vi "run.description.vi"(8 "error in":errorcluster, 11 "Run in":refnum<class "Run.lvclass">) -> (0 "error out":errorcluster, 3 "Run out":refnum<class "Run.lvclass">)   [LabVIEW 2020, in "Run.lvclass"]
doc: "Returns the run's description."
uses:
  Run.lvclass
  Run.lvclass/Run.ctl
  client.lvlib
panel:
  out "out_needed out":u32
  out "description":string
  in  "buf":string
  in  "cap":u32
  in  "out_needed":u32
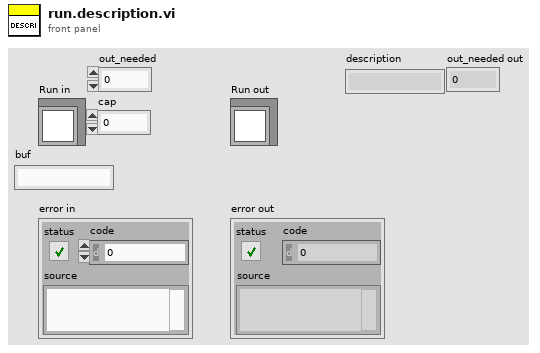
[diagram p1: front panel]
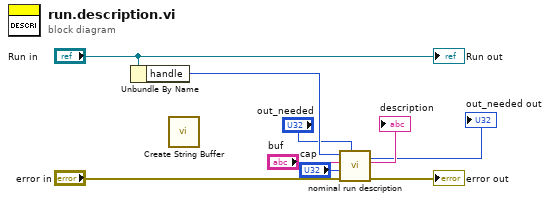
[diagram p0: block diagram]
diagram:
  n1 = Unbundle By Name("Run in") -> ("handle"=w7:i32)
  n2 = call "Create String Buffer.vi"() -> ()  [unwired: 9 in, 3 out]
  n3 = call "nominal run description.vi"("out_needed"="out_needed", "error in (no error)"="error in", "cap"="cap", "buf"="buf", "run"=w7) -> ("error out"=→"error out":errorcluster, "buf out"=→"description":string, "out_needed out"=→"out_needed out":u32)  [unwired: 3 in, 1 out]
  "Run out" <- "Run in"
